vi "Set Sessions_niVNA.vi"(11 "Semiconductor Module Context":T1) -> (0 "error out":errorcluster)   [LabVIEW 2013]
uses:
  <vilib>/NI_TestStand_SemiconductorModule/NI_TestStand_Semiconductor_Module.lvlibp/PinMap/General/SemiconductorModuleContext.ctl
  <vilib>/NI_TestStand_SemiconductorModule/NI_TestStand_Semiconductor_Module.lvlibp
  VNA/Pin Map API/VNA Custom Instrument.lvlib
  DMM/Pin Map API/DMM Custom Instruments.lvlib
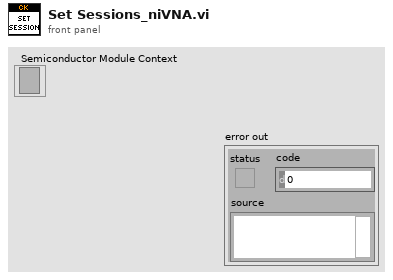
[diagram p1: front panel]
types:
  T1 = typedef "NI_TestStand_Semiconductor_Module.lvlibp/SemiconductorModuleContext.ctl" = refnum<k7>
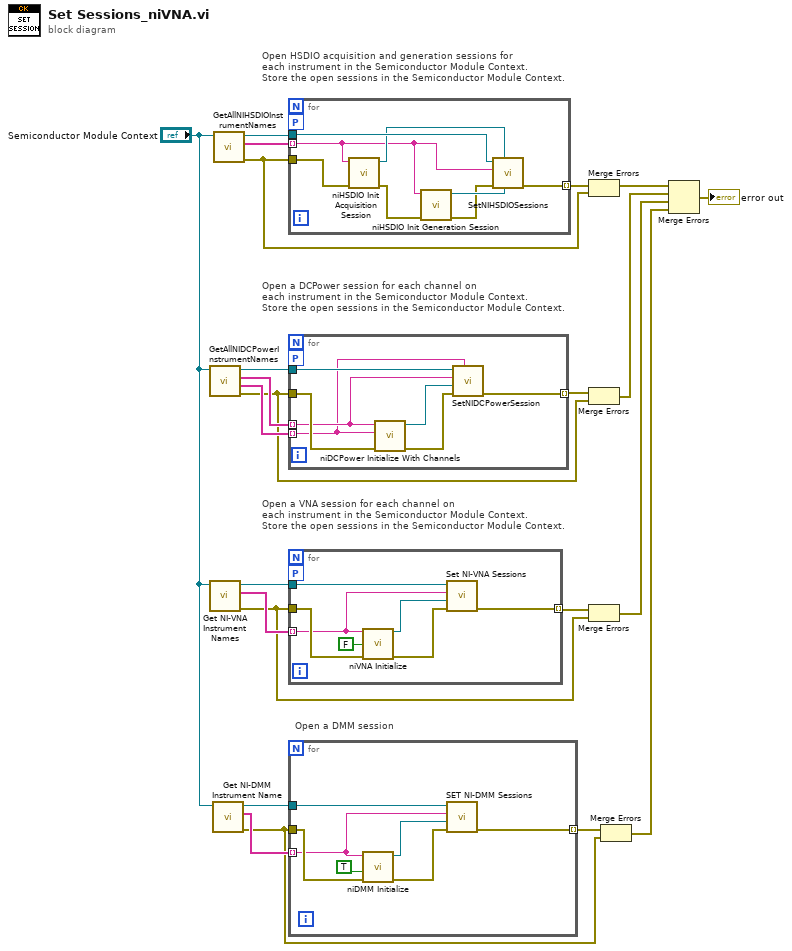
[diagram p0: block diagram]
diagram:
  # "Open a DMM session"
  # "Open a VNA session for each channel on \neach instrument in the Semiconductor Module Context.\nStore the open sessions in the Semiconductor Module Context."
  # "Open a DCPower session for each channel on \neach instrument in the Semiconductor Module Context.\nStore the open sessions in the Semiconductor Module Context."
  # "Open HSDIO acquisition and generation sessions for\neach instrument in the Semiconductor Module Context.\nStore the open sessions in the Semiconductor Module Context."
  n1 = call <vilib>:"GetAllNIDCPowerInstrumentNames.vi"("Semiconductor Module Context"="Semiconductor Module Context") -> ("error out"=w10:errorcluster, "Channel Ids"=w19:string[], "Instrument Names"=w22:string[], "Semiconductor Module Context Out"=w21:T1)  [unwired: 7 in]
  n2 = call "Get NI-VNA Instrument Names.vi"("Semiconductor Module Context"="Semiconductor Module Context") -> ("error out"=w13:errorcluster, "Instrument Names"=w17:string[], "Semiconductor Module Context Out"=w16:T1)  [unwired: 7 in, 1 out]
  n3 = call "Get NI-DMM Instrument Name.vi"("Semiconductor Module Context"="Semiconductor Module Context") -> ("Semiconductor Module Context Out"=w6:T1, "Instrument Names"=w5:string[], "error out"=w3:errorcluster)  [unwired: 6 in, 1 out]
  n4 = call <vilib>:"GetAllNIHSDIOInstrumentNames.vi"("Semiconductor Module Context"="Semiconductor Module Context") -> ("error out"=w7:errorcluster, "Instrument Names"=w23:string[], "Semiconductor Module Context Out"=w18:T1)  [unwired: 8 in]
  n5 = for {
    tunnel: w23 -> [w25] mode=indexing
    tunnel: w7 -> [w31]
    tunnel: [w27] -> w8 mode=indexing
    tunnel: w18 -> [w30]
    workers-P: _ -> [_]
    n6 = call <instrlib>:"niHSDIO Init Acquisition Session.vi"("error in (no error)"=w31, "resource name"=w25) -> ("error out"=w26:errorcluster, "instrument handle out"=w29:refnum<k15>)  [unwired: 8 in]
    n7 = call <instrlib>:"niHSDIO Init Generation Session.vi"("error in (no error)"=w26, "resource name"=w25) -> ("error out"=w24:errorcluster, "instrument handle out"=w28:refnum<k15>)  [unwired: 8 in]
    n8 = call <vilib>:"SetNIHSDIOSessions.vi"("Generation Session"=w28, "Acquisition Session"=w29, "error in (no error)"=w24, "Instrument Name"=w25, "Semiconductor Module Context"=w30) -> ("error out"=w27:errorcluster)  [unwired: 5 in, 1 out]
  }
  n9 = for {
    tunnel: w22 -> [w35] mode=indexing
    tunnel: w19 -> [w32] mode=indexing
    workers-P: _ -> [_]
    tunnel: w10 -> [w36]
    tunnel: [w37] -> w12 mode=indexing
    tunnel: w21 -> [w38]
    n10 = call <instrlib>:"niDCPower Initialize With Channels.vi"("error in (no error)"=w36, "channels"=w32, "resource name"=w35) -> ("error out"=w34:errorcluster, "instrument handle out"=w33:refnum<k15>)  [unwired: 7 in]
    n11 = call <vilib>:"SetNIDCPowerSession.vi"("Channel Id"=w32, "error in (no error)"=w34, "Instrument Session"=w33, "Instrument Name"=w35, "Semiconductor Module Context"=w38) -> ("error out"=w37:errorcluster)  [unwired: 5 in, 1 out]
  }
  n12 = for {
    tunnel: w17 -> [w40] mode=indexing
    workers-P: _ -> [_]
    tunnel: w13 -> [w45]
    tunnel: [w42] -> w15 mode=indexing
    tunnel: w16 -> [w43]
    n13 = call <instrlib>:"niVNA Initialize.vi"("resource name"=w40, "reset"=FALSE, "error in"=w45) -> ("instrument handle"=w41:refnum<k15>, "error out"=w44:errorcluster)  [unwired: 11 in]
    n14 = call "Set NI-VNA Sessions.vi"("error in (no error)"=w44, "Instrument Session"=w41, "Instrument Name"=w40, "Semiconductor Module Context"=w43) -> ("error out"=w42:errorcluster)  [unwired: 6 in, 1 out]
  }
  n15 = for {
    tunnel: w5 -> [w48] mode=indexing
    tunnel: w6 -> [w50]
    tunnel: w3 -> [w52]
    tunnel: [w49] -> w4 mode=indexing
    n16 = call <instrlib>:"niDMM Initialize.vi"("error in (no error)"=w52, "Reset"=TRUE ("ID Query"), "Instrument Descriptor"=w48) -> ("error out"=w51:errorcluster, "instrument handle out"=w47:refnum<k15>)  [unwired: 7 in]
    n17 = call "SET NI-DMM Sessions.vi"("error in (no error)"=w51, "Instrument Session"=w47, "Instrument Name"=w48, "Semiconductor Module Context"=w50) -> ("error out"=w49:errorcluster)  [unwired: 6 in, 1 out]
  }
  n18 = Merge Errors(w8, w7) -> (w9:errorcluster)
  n19 = Merge Errors(w12, w10) -> (w11:errorcluster)
  n20 = Merge Errors(w15, w13) -> (w14:errorcluster)
  n21 = Merge Errors(w4, w3) -> (w2:errorcluster)
  n22 = Merge Errors(w9, w11, w14, w2) -> (→"error out":errorcluster)
